vi "tabenableProperty.vi"() -> ()   [LabVIEW 2021]
panel:
  in  "Slide":dbl(slide) scale=0.0..10.0
  in  "Tab Control":enum32{"Page 1", "Page 2"}(tab)
  in  "Thermometer":dbl(slide) scale=0.0..100.0
  in  "Boolean":bool
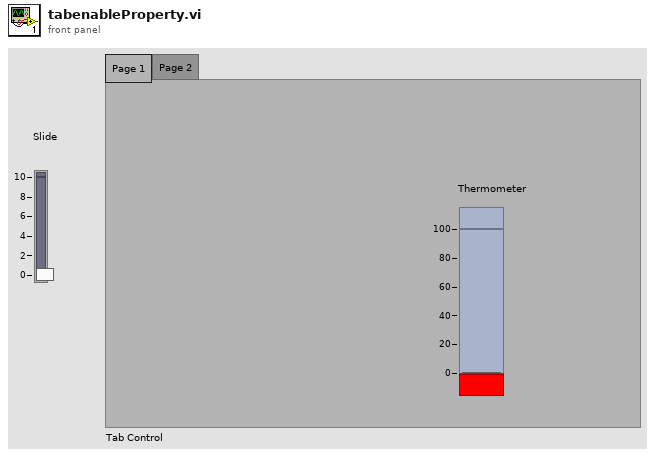
[diagram p1: front panel]
types:
  T1 = enum32{"Page Enabled", "Page Disabled", "Page Disabled & Grayed"}
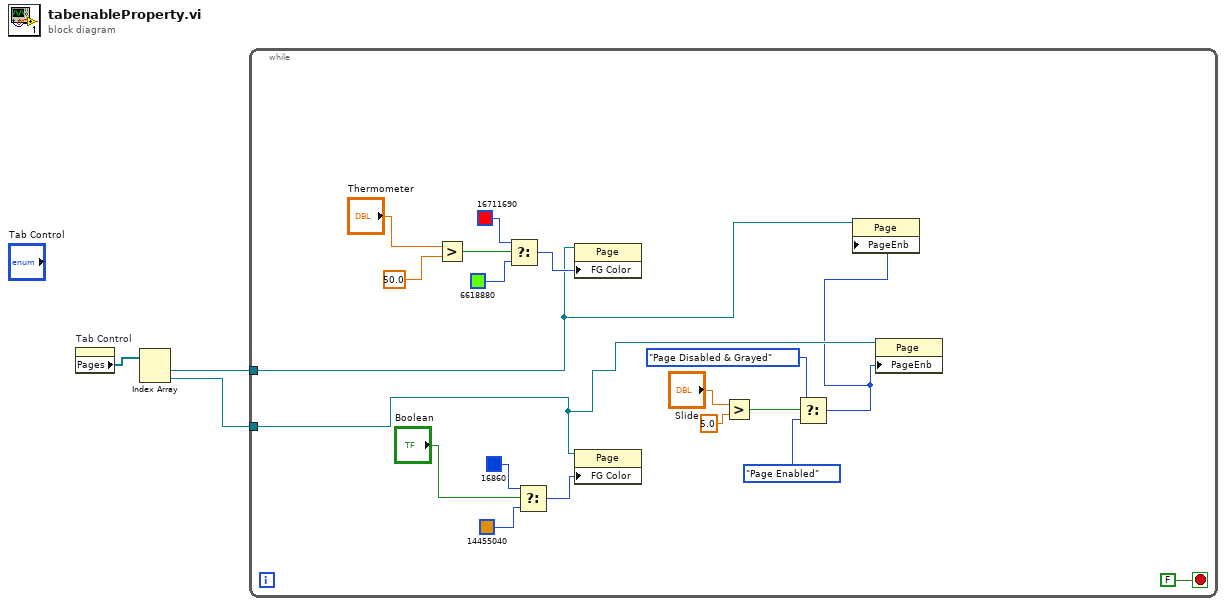
[diagram p0: block diagram]
diagram:
  n1 = property on="Tab Control" class="TabCtl (strict)"() -> ("Pages"=w3:refnum<vi>[])  [unwired: 2 in, 2 out]
  n2 = Index Array(array=w3) -> (element #1=w2:refnum<vi>, element #2=w1:refnum<vi>)  [unwired: 2 in]
  n3 = while {
    tunnel: w2 -> [w4]
    tunnel: w1 -> [w8]
    stop <- FALSE stop-if-true
    n4 = Greater?(x="Thermometer", y=50.0) -> (0:w19:bool)
    n5 = Select(t=u32 16711690 ("Color Box"), s=w19, f=u32 6618880 ("Color Box")) -> (s? t:f=w16:u32)
    n6 = Select(t=u32 16860 ("Color Box"), s="Boolean", f=u32 14455040 ("Color Box")) -> (s? t:f=w13:u32)
    n7 = property class="Page"(reference=w4, "FG Color"=w16) -> ()  [unwired: 1 in, 2 out]
    n8 = property class="Page"(reference=w8, "FG Color"=w13) -> ()  [unwired: 1 in, 2 out]
    n9 = Greater?(x="Slide", y=5.0) -> (0:w9:bool)
    n10 = Select(t=T1."Page Disabled & Grayed" ("Page Enabled State"), s=w9, f=T1."Page Enabled" ("Page Enabled State")) -> (s? t:f=w5:T1)
    n11 = property class="Page"(reference=w4, "PageEnb"=w5) -> ()  [unwired: 1 in, 2 out]
    n12 = property class="Page"(reference=w8, "PageEnb"=w5) -> ()  [unwired: 1 in, 2 out]
  }
